vi "Get Queues.vi"(8 "error in (no error)":errorcluster, 11 "Test Redis Client in":refnum<class "Test Redis Client.lvclass">) -> (0 "error out":errorcluster, 1 "receive queue":refnum<queue>, 2 "send queue":refnum<queue>, 3 "Test Redis Client out":refnum<class "Test Redis Client.lvclass">)   [LabVIEW 2019, in "Test Redis Client for LabVIEW.lvlib" / "Test Redis Client.lvclass"]
uses:
  Test Redis Client.lvclass
  Test Redis Client.lvclass/Test Redis Client.ctl
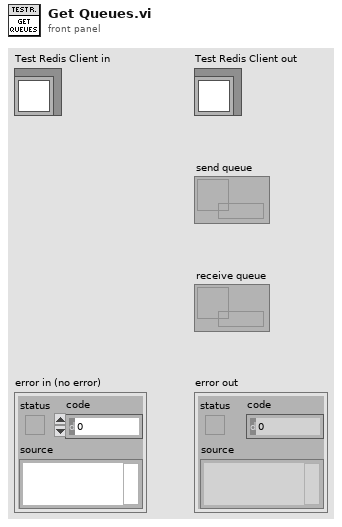
[diagram p1: front panel]
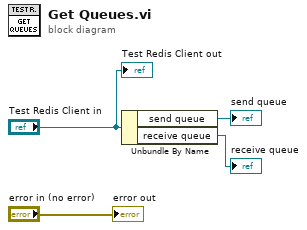
[diagram p0: block diagram]
diagram:
  n1 = Unbundle By Name("Test Redis Client in") -> ("send queue"=→"send queue":refnum<queue>, "receive queue"=→"receive queue":refnum<queue>)
  "error out" <- "error in (no error)"
  "Test Redis Client out" <- "Test Redis Client in"
